vi "UsrProfiles-Save user profile-with dialogue.vi"   [LabVIEW 2013]
uses:
  Typedefs/Which path.ctl
  Globals/gl_UsrProfiles globals.vi
types:
  T1 = typedef "Which path.ctl" = enum16{"Configuration Files", "Calibration Files", "Images", "Setup.ini", "Loaded User profile.ini", "User's-Previous session.ini", "New user profile.ini", "Selected User profile.ini", "User profiles folder", "Power meter scaling.txt", "FOV Cal.ini"}
  T2 = typedef "Button Pressed.ctl" = enum16{"Left button", "Middle button", "Right button"}
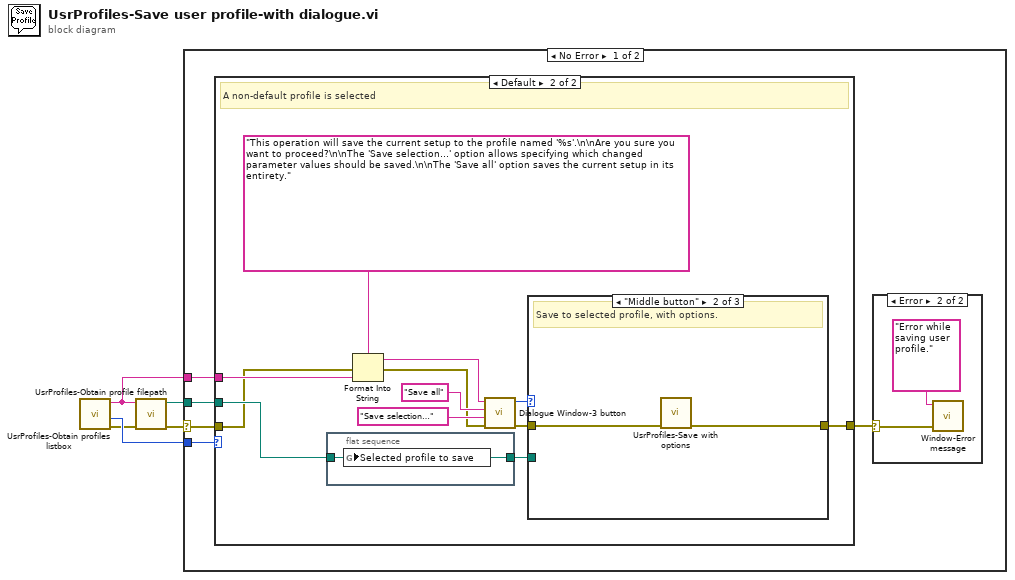
[diagram p0: block diagram]
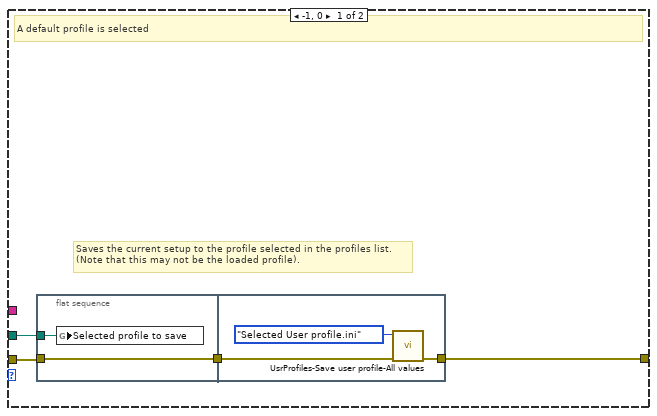
[diagram p3: hidden frame]
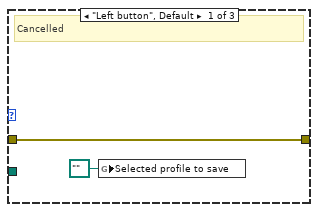
[diagram p4: hidden frame]
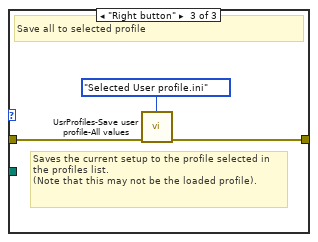
[diagram p5: hidden frame]
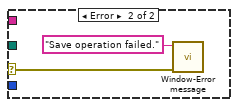
[diagram p6: hidden frame]
diagram:
  n1 = call "UsrProfiles-Obtain profiles listbox.vi"() -> ("error out"=w3:errorcluster, "Selection's index"=w5:i32, "Selected profile's name"=w4:string)  [unwired: 8 in, 1 out]
  n2 = call "UsrProfiles-Obtain profile filepath.vi"("error in"=w3, "Profile name"=w4) -> ("error out"=w2:errorcluster, "Profile filepath"=w1:path)  [unwired: 8 in]
  n3 = case shown="No Error" w2 {
    selector: w2 -> [w7 w43]
    tunnel: w5 -> [w10 _]
    tunnel: w4 -> [w9 _]
    tunnel: w1 -> [w8 _]
    frame No Error {
      n4 = case shown="Default" w10 {
        tunnel: w9 -> [_ w28]
        tunnel: w7 -> [w14 w25]
        tunnel: w8 -> [w16 w27]
        tunnel: [w13 w22] -> w6
        frame -1, 0 {
          # "Saves the current setup to the profile selected in the profiles list.\n(Note that this may not be the loaded profile)."
          # "A default profile is selected"
          n5 = flat-sequence {
            tunnel: w16 -> [w18]
            tunnel: [w17] -> w15
            tunnel: w14 -> [w17]
            tunnel: w15 -> [w20]
            tunnel: [w19] -> w13
            frame #0 {
              n6 = global write "gl_UsrProfiles globals.vi" "Selected profile to save"(w18) -> ()
            }
            frame #1 {
              n7 = call "UsrProfiles-Save user profile-All values.vi"("error in"=w20, "Which file? (User profile.ini)"=Which_path."Selected User profile.ini") -> ("error out"=w19:errorcluster)  [unwired: 9 in]
            }
          }
        }
        frame Default {
          # "A non-default profile is selected"
          n8 = flat-sequence {
            tunnel: w27 -> [w34]
            tunnel: [w34] -> w26
            frame #0 {
              n9 = global write "gl_UsrProfiles globals.vi" "Selected profile to save"(w34) -> ()
            }
          }
          n10 = Format Into String(format string="This operation will save the current setup to the profile named '%s'.\n\nAre you sure you want to proceed?\n\nThe 'Save selection…' option allows specifying which changed parameter values should be saved.\n\nThe 'Save all' option saves the current setup in its entirety." ("Message string"), error in=w25, w28) -> (resulting string=w31:string, error out=w24:errorcluster)  [unwired: 1 in]
          n11 = call "Dialogue Window-3 button.vi"("error in (no error)"=w24, "Caption-Middle button"="Save selection…", "Caption-Right button (OK)"="Save all", "Message string"=w31) -> ("error out"=w23:errorcluster, "Button pressed"=w32:T2)  [unwired: 5 in, 1 out]
          n12 = case shown="\"Middle button\"" w32 {
            tunnel: w26 -> [_ _ _]
            tunnel: w23 -> [w36 w38 w40]
            tunnel: [w36 w37 w39] -> w22
            frame "Left button", Default {
              # "Cancelled"
              n13 = global write "gl_UsrProfiles globals.vi" "Selected profile to save"(path "" ("Selected profile to save")) -> ()
            }
            frame "Middle button" {
              # "Save to selected profile, with options."
              n14 = call "UsrProfiles-Save with options.vi"("error in"=w38) -> ("error out"=w37:errorcluster)  [unwired: 10 in]
            }
            frame "Right button" {
              # "Saves the current setup to the profile selected in the profiles list.\n(Note that this may not be the loaded profile)."
              # "Save all to selected profile"
              n15 = call "UsrProfiles-Save user profile-All values.vi"("error in"=w40, "Which file? (User profile.ini)"=Which_path."Selected User profile.ini") -> ("error out"=w39:errorcluster)  [unwired: 9 in]
            }
          }
        }
      }
      n16 = case shown="Error" w6 {
        selector: w6 -> [_ w12]
        frame No Error {
        }
        frame Error {
          n17 = call "Window-Error message.vi"("error in (no error)"=w12, "Message"="Error while saving user profile.") -> ()  [unwired: 9 in, 1 out]
        }
      }
    }
    frame Error {
      n18 = call "Window-Error message.vi"("error in (no error)"=w43, "Message"="Save operation failed.") -> ()  [unwired: 9 in, 1 out]
    }
  }
